vi "SampleCalibrationLoadPlate.vi"(8 "Error In":errorcluster, 11 "MotorController in":refnum<class "MotorController.lvclass">) -> (0 "Error Out":errorcluster, 3 "MotorController out":refnum<class "MotorController.lvclass">)   [LabVIEW 2019]
uses:
  MotorController.lvclass
panel:
  in  "Next":bool
  # "Sample Calibration - Install Grid Plate"
  # "Install the grid plate once the machine has moved to the load position."
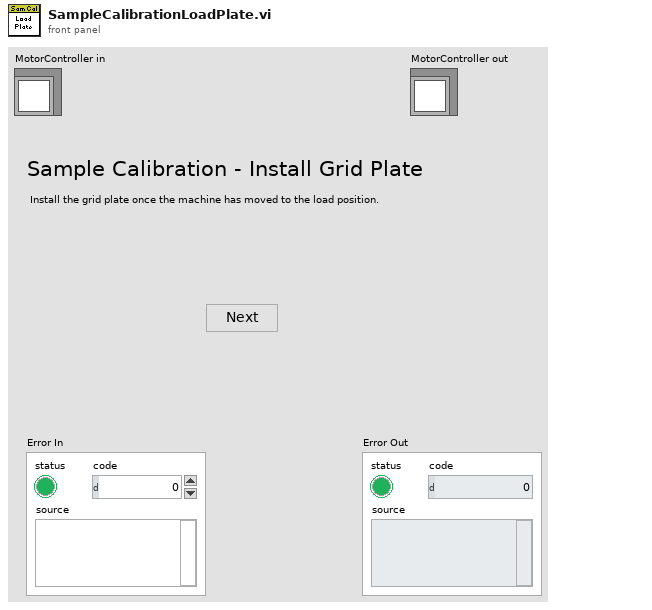
[diagram p1: front panel]
types:
  T1 = enum8{"Enabled", "Disabled", "Disabled and Grayed Out"}
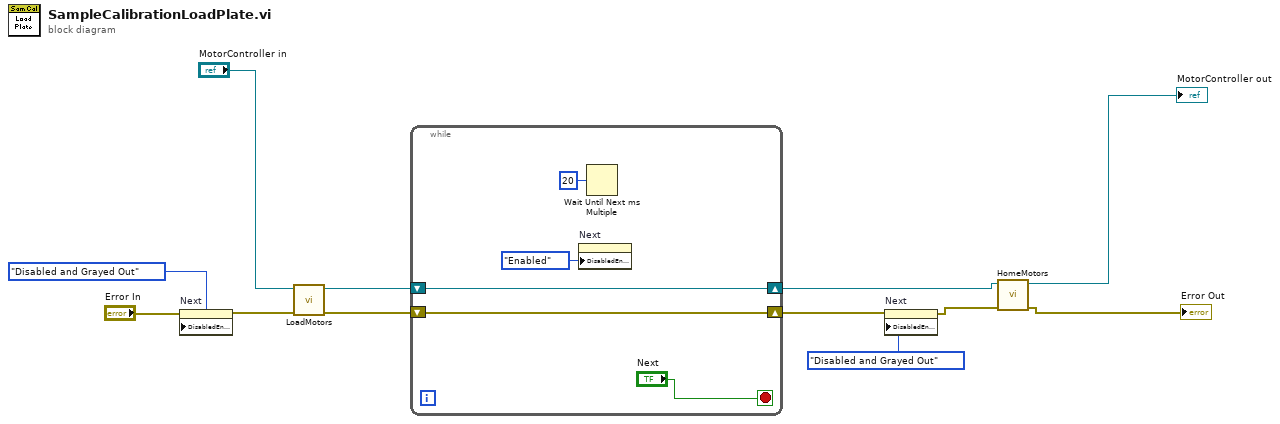
[diagram p0: block diagram]
diagram:
  n1 = property on="Next" class="Bool"(error in="Error In", "DisabledEnum"=T1."Disabled and Grayed Out" ("Disabled")) -> (error out=w10:errorcluster)  [unwired: 1 in, 1 out]
  n2 = call "LoadMotors.vi"("error in (no error)"=w10, "MotorController in"="MotorController in") -> ("error out"=w8:errorcluster, "MotorController out"=w7:refnum<class "MotorController.lvclass">)  [unwired: 8 in]
  n3 = while {
    shift-right: [w15] -> w5
    shift-left: w8 -> [w15]
    shift-right: [w13] -> w4
    shift-left: w7 -> [w13]
    stop <- "Next" stop-if-true
    n4 = property on="Next" class="Bool"("DisabledEnum"=T1."Enabled" ("Disabled")) -> ()  [unwired: 2 in, 2 out]
    n5 = Wait Until Next ms Multiple(millisecond multiple=u32 20) -> ()  [unwired: 1 out]
  }
  n6 = property on="Next" class="Bool"(error in=w5, "DisabledEnum"=T1."Disabled and Grayed Out" ("Disabled")) -> (error out=w3:errorcluster)  [unwired: 1 in, 1 out]
  n7 = call "HomeMotors.vi"("error in (no error)"=w3, "MotorController in"=w4) -> ("error out"=→"Error Out":errorcluster, "MotorController out"=→"MotorController out":refnum<class "MotorController.lvclass">)  [unwired: 8 in]
